vi "Test_sqlite3ListTables_ListsTables.vi"(8 "error in (no error)":errorcluster, 11 "TestCase in":refnum<class "Test sqlite3.lvclass">) -> (0 "error out":errorcluster, 3 "TestCase out":refnum<class "Test sqlite3.lvclass">)   [LabVIEW 2020, in "Test sqlite3.lvclass"]
uses:
  Test sqlite3.lvclass
  Test sqlite3.lvclass/Test sqlite3.ctl
  externals/sqlite3/Source/sqlite3.lvclass
  <vilib>/addons/_JKI Toolkits/VI Tester/TestCase.llb/TestCase.lvclass
  C:/Program Files/National Instruments/LabVIEW 2020/vi.lib/addons/_JKI Toolkits/VI Tester/TestCase.llb/TestCase.lvclass
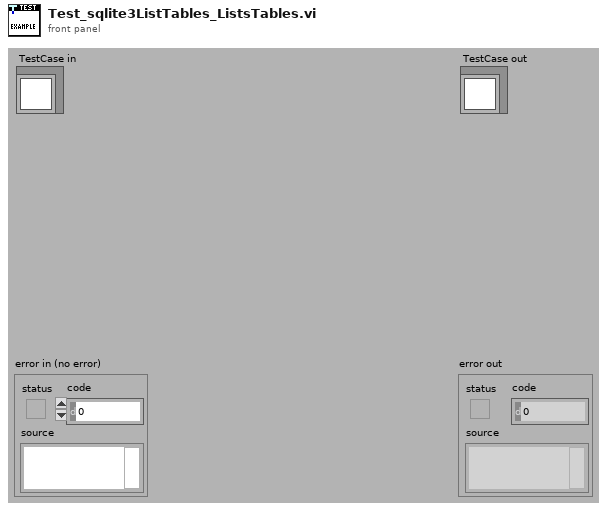
[diagram p1: front panel]
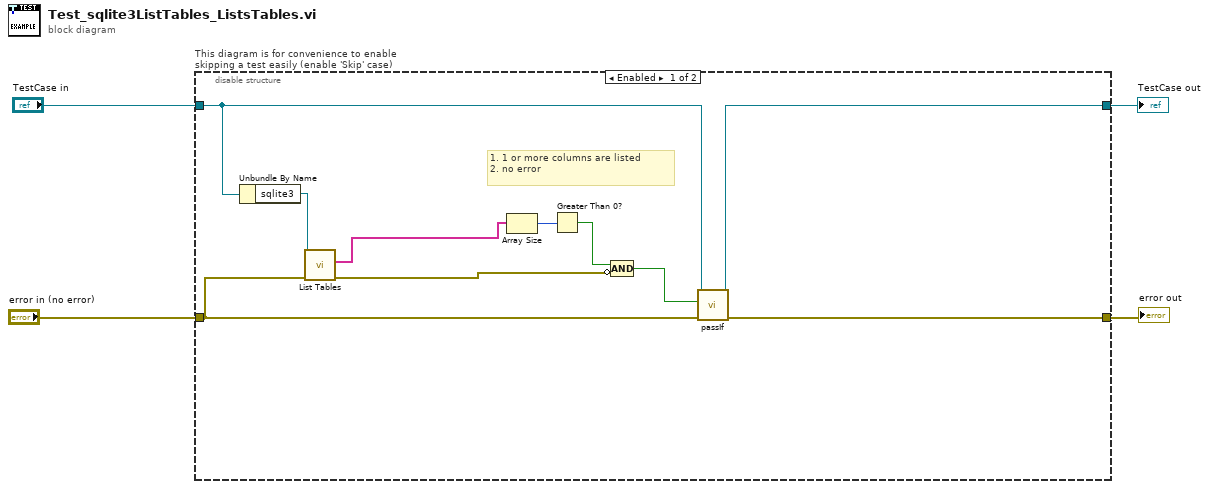
[diagram p0: block diagram]
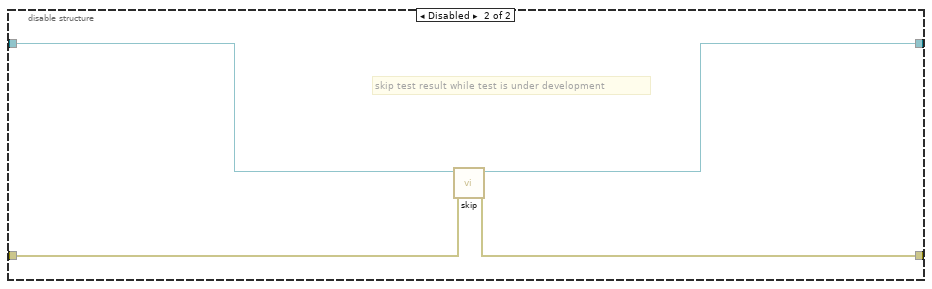
[diagram p2: hidden frame]
diagram:
  n1 = disable-structure "This diagram is for convenience to enable skipping a test easily (enable 'Skip' case)" shown="Enabled" {
    disable-tunnel: "TestCase in" -> [w12 w18]
    disable-tunnel: [w14 w16] -> w1
    disable-tunnel: [w13 w17] -> w3
    disable-tunnel: "error in (no error)" -> [w10 w15]
    frame Enabled {
      # "1. 1 or more columns are listed\n2. no error"
      n2 = Unbundle By Name(w12) -> ("sqlite3"=w11:refnum<class "sqlite3.lvclass">)
      n3 = call-dynamic "List Tables.vi"("error in (no error)"=w10, "sqlite in"=w11) -> ("error out"=w6:errorcluster, "Tables out"=w5:string[])  [unwired: 7 in, 1 out]
      n4 = Array Size(array=w5) -> (size(s)=w9:i32)
      n5 = Greater Than 0?(x=w9) -> (x > 0?=w8:bool)
      n6 = Compound Arithmetic op=AND(w8, invert w6) -> (w7:bool)
      n7 = call-dynamic "passIf.vi"("error in (no error)"=w10, "pass"=w7, "TestCase in"=w12) -> ("error out"=w13:errorcluster, "TestCase out"=w14:refnum<class "Test sqlite3.lvclass">)  [unwired: 7 in]
    }
    frame Disabled {
      # "skip test result while test is under development"
      n8 = call <vilib>:"skip.vi"("error in (no error)"=w15, "TestCase in"=w18) -> ("error out"=w17:errorcluster, "TestCase out"=w16:refnum<class "Test sqlite3.lvclass">)  [unwired: 8 in]
    }
  }
  "error out" <- w3
  "TestCase out" <- w1
